vi "Process.vi"(8 "error in":errorcluster, 11 "EmbeddedMainUI":refnum<class "EmbeddedMainUI.lvclass">) -> (0 "error out":errorcluster, 3 "EmbeddedMainUI out":refnum<class "EmbeddedMainUI.lvclass">)   [LabVIEW 2016, in "EmbeddedMainUI.lvclass"]
doc: "---------------------------------------------------------------\nJKI State Machine Objects™\nhttp://jki.net/state-machine-objects/\nCopyright (C) 2005-2015, JKI <info@jki.net>\nALL RIGHTS RESERVEDJKI State Machine Objects (SMO) 1.0.0.5\nJKI - JKI\nCopyright (c) 2016, JKI"
uses:
  EmbeddedMainUI.lvclass
  C:/Program Files (x86)/National Instruments/LabVIEW 2016/vi.lib/JKI/JKI SMO/SMO/SMO.lvclass
  C:/Program Files (x86)/National Instruments/LabVIEW 2016/vi.lib/JKI/JKI SMO/SMO.UI/SMO.UI.lvclass
  <vilib>/JKI/JKI SMO/SMO/Typedefs/Parent Call--Enum.ctl
  <vilib>/Levylab/Embedded SMO UI/EmbeddedSMO.lvclass
  <vilib>/JKI/JKI SMO/SMO.UI/SMO.UI.lvclass
  <vilib>/JKI/JKI SMO/SMO/SMO.lvclass
panel:
  in  "Right Ring":u16(ring) items=["State One"]
  in  "Left Ring":u16(ring) items=["Mock1", "Mock2", "Mock3"]
  # "For instructions on how to use the JKI State Machine Objects, examples and video tutorials, visit:\nhttp://jki.net/state-machine-objects/\n\nJKI State Machine Objects™\nhttp://jki.net/state-machine-objects/\nCopyright (C) 2005-2015, JKI <info@jki.net>\nALL RIGHTS RESERVED"
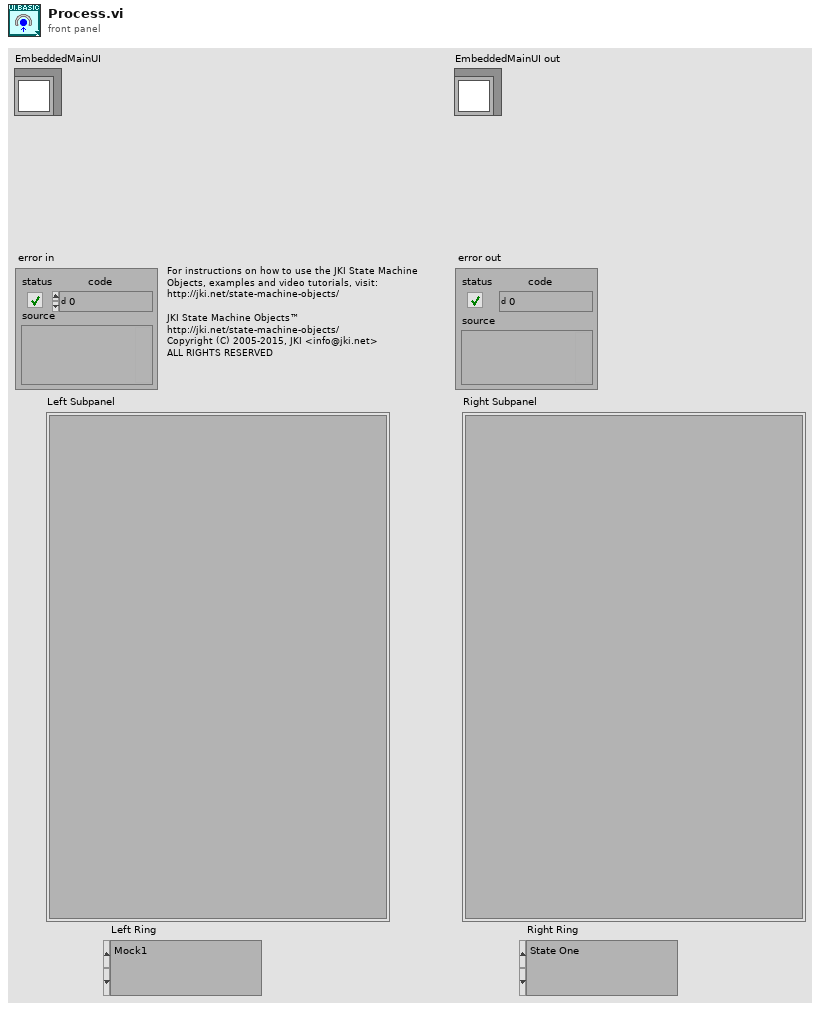
[diagram p1: front panel]
types:
  T1 = typedef "SMO.lvclass/Parent Call--Enum.ctl" = enum16{"Allows parent to run", "Does not request parent to run"}
  T2 = enum32{"invalid app kind", "Development System", "Run Time System", "Student Edition", "Embedded LabVIEW", "Evaluation", "Custom"}
  T3 = enum32{"Invalid", "Standard", "Closed", "Hidden", "Minimized", "Maximized"}
  T4 = cluster{"Core":cluster{"Current VI Reference":refnum<vi>, "Close Panel on Exit?":bool, "error":errorcluster}, "Self Reference":refnum<class "EmbeddedMainUI.lvclass">, "Right Subpanel":refnum<vi>, "Left Subpanel":refnum<vi>, "Left Ring":refnum<vi>, "Right Ring":refnum<vi>}
  T5 = cluster{"Current VI Reference":refnum<vi>, "Close Panel on Exit?":bool, "error":errorcluster}
  T6 = typedef "SMO.lvclass/Protected Events.ctl" = cluster{"StopProcesses":refnum<user-event>, "AbortProcesses":refnum<user-event>, "Config Changed":refnum<user-event>, "Dependency":refnum<user-event>}
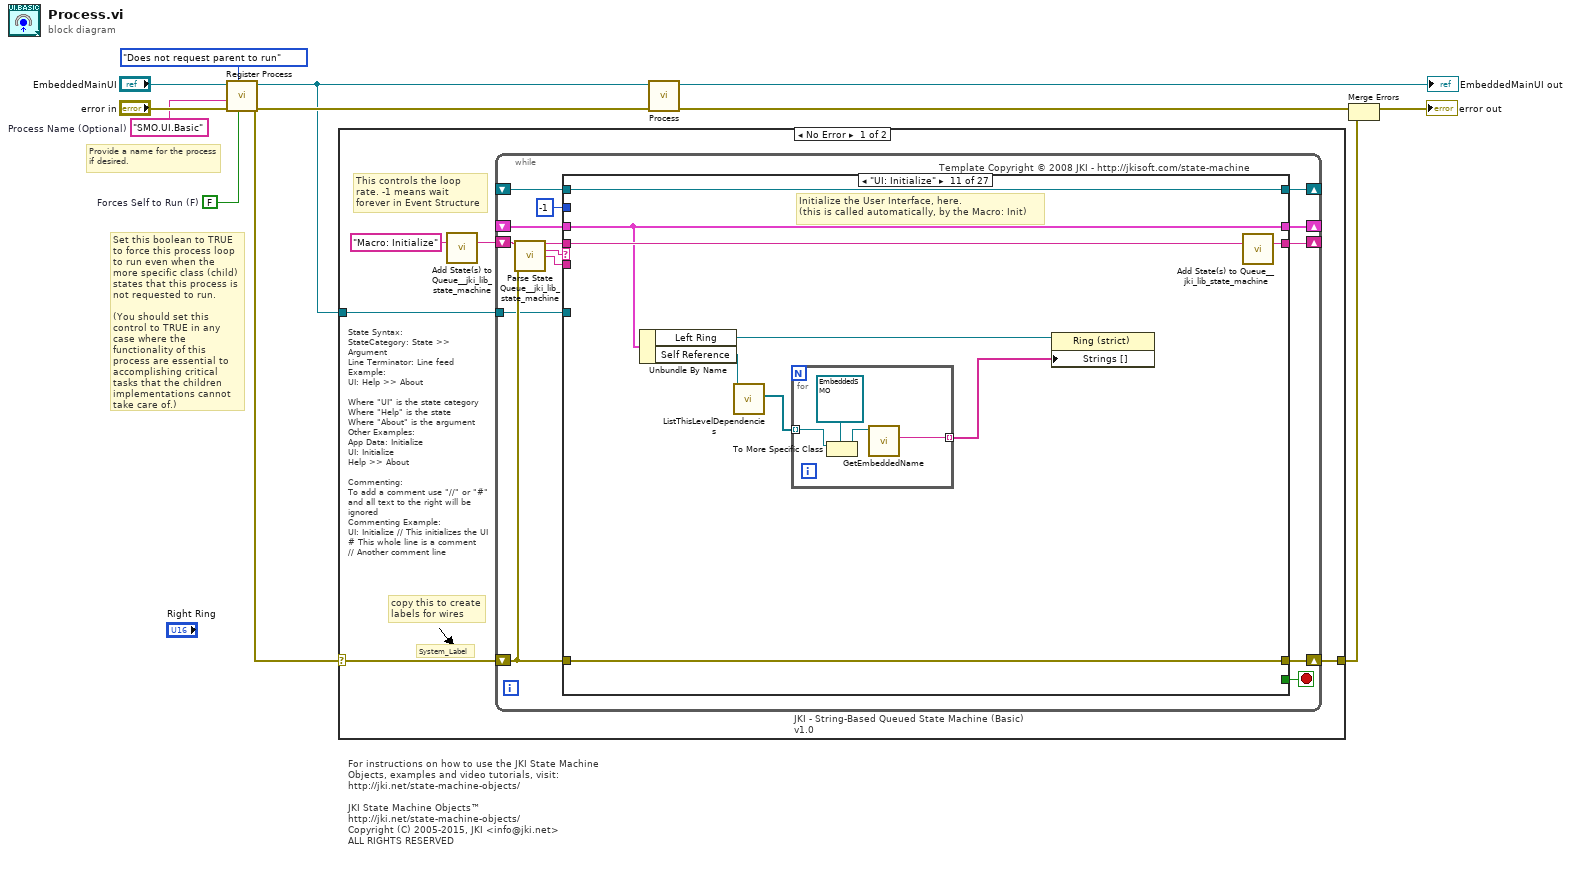
[diagram p0: block diagram]
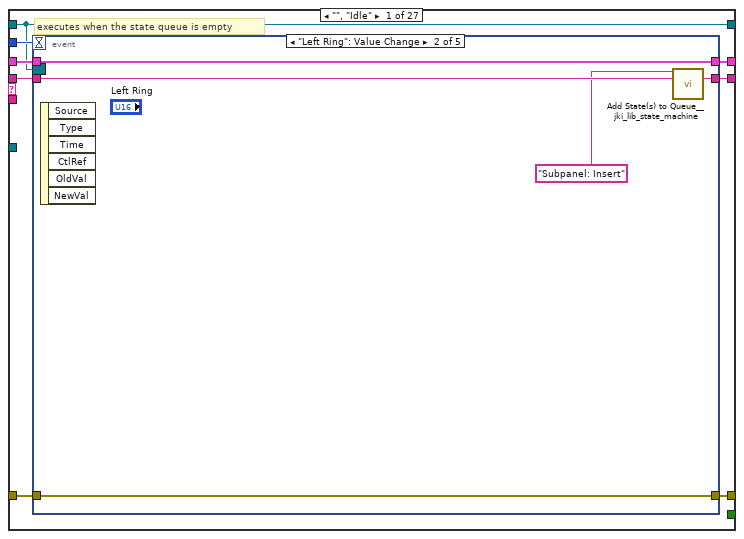
[diagram p2: hidden frame]
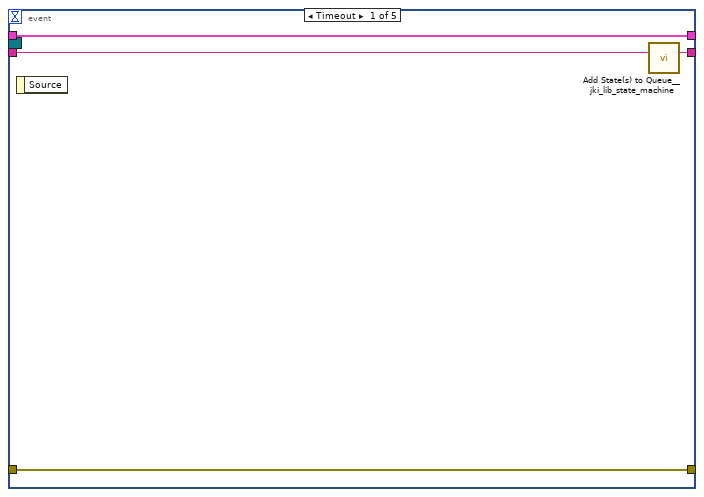
[diagram p3: hidden frame]
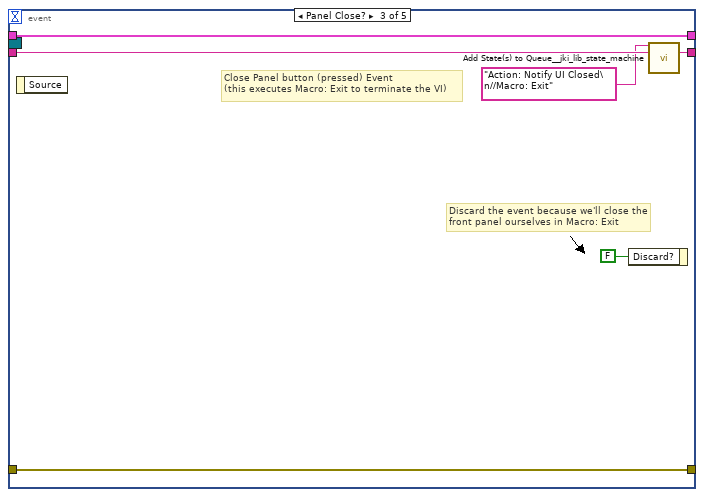
[diagram p4: hidden frame]
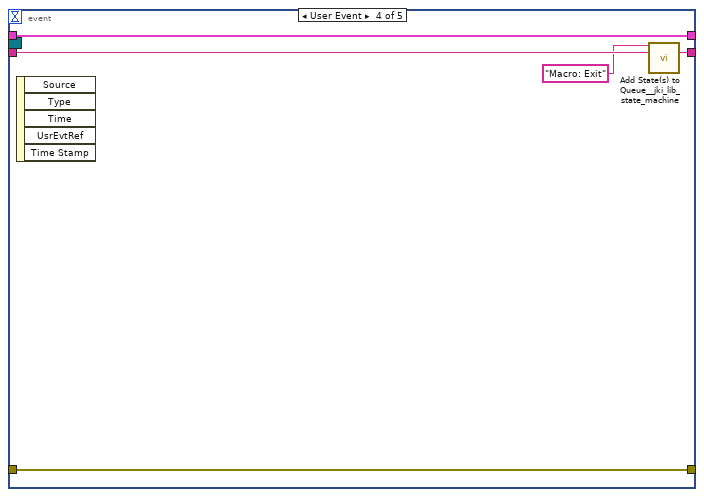
[diagram p5: hidden frame]
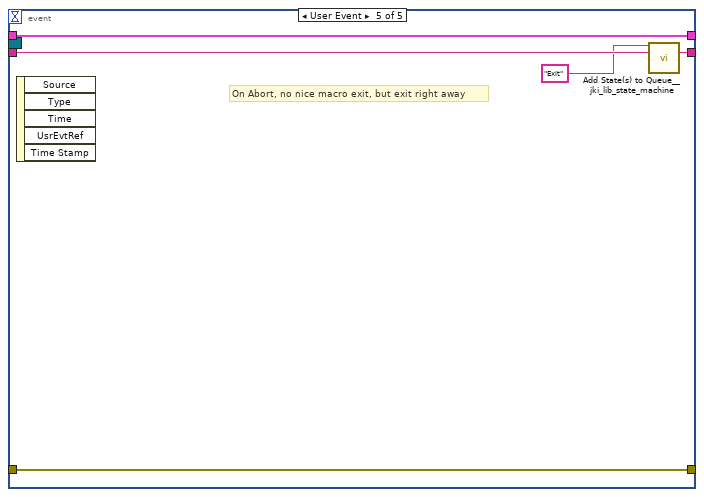
[diagram p6: hidden frame]
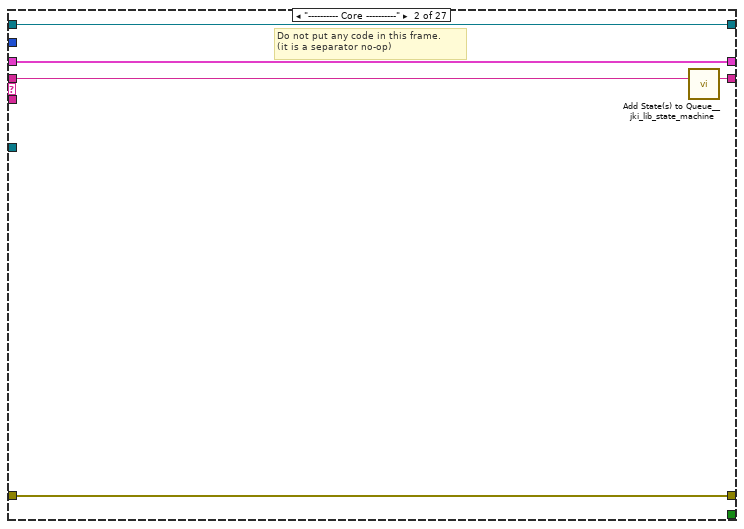
[diagram p7: hidden frame]
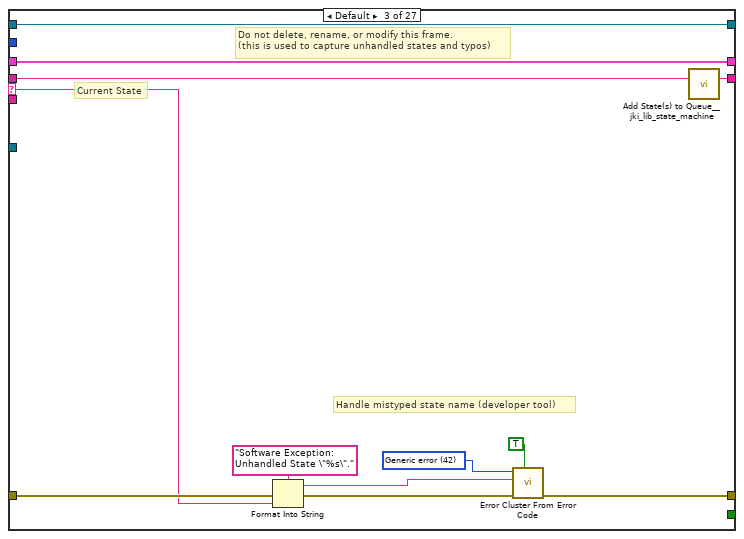
[diagram p8: hidden frame]
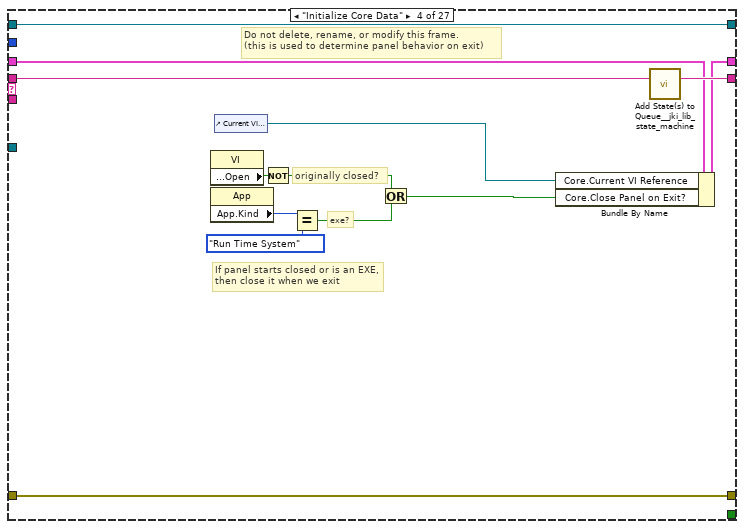
[diagram p9: hidden frame]
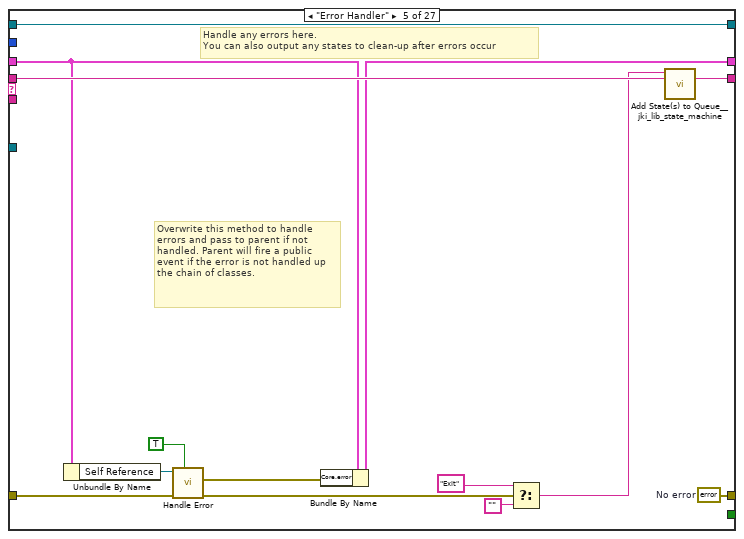
[diagram p10: hidden frame]
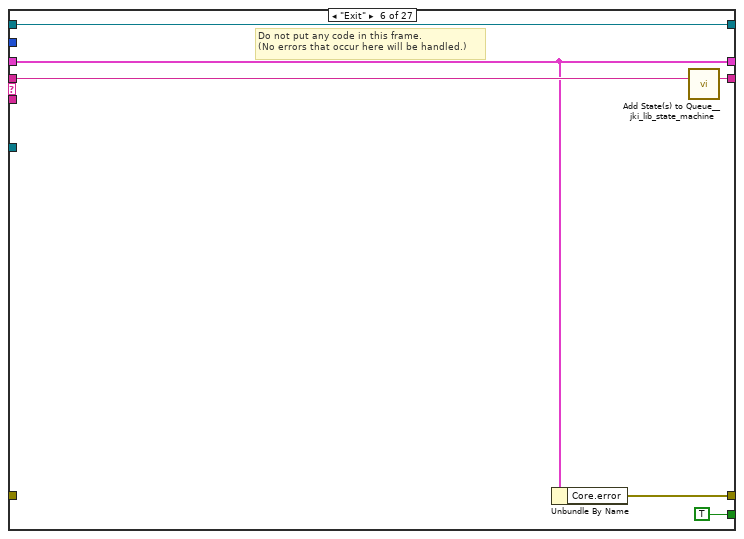
[diagram p11: hidden frame]
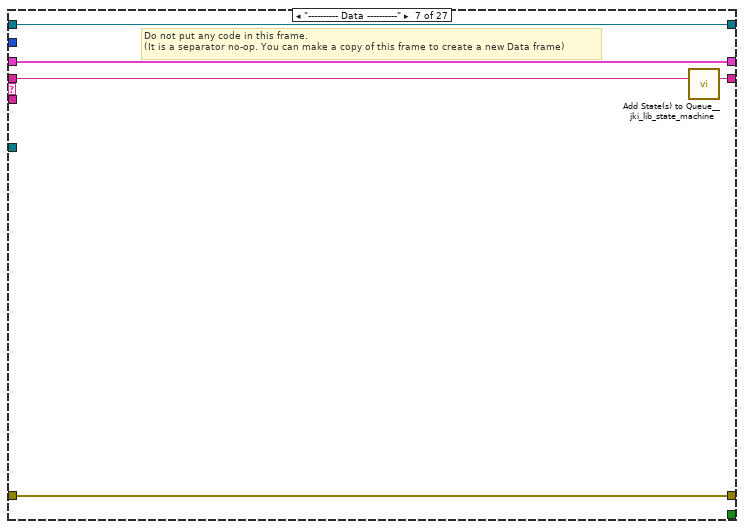
[diagram p12: hidden frame]
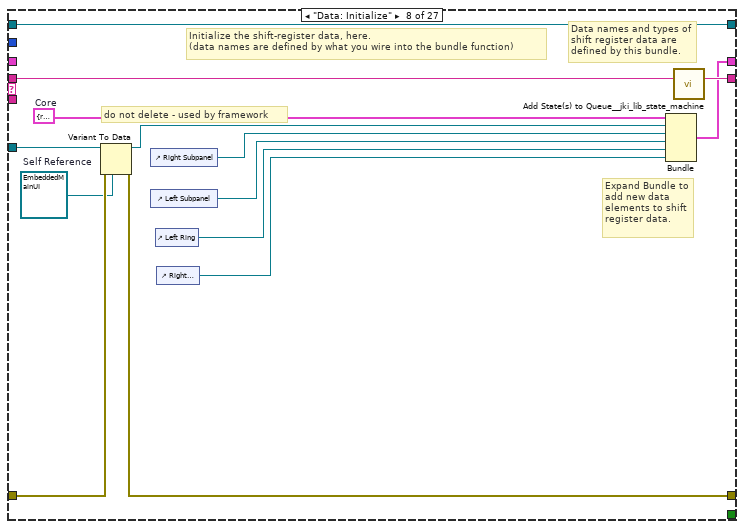
[diagram p13: hidden frame]
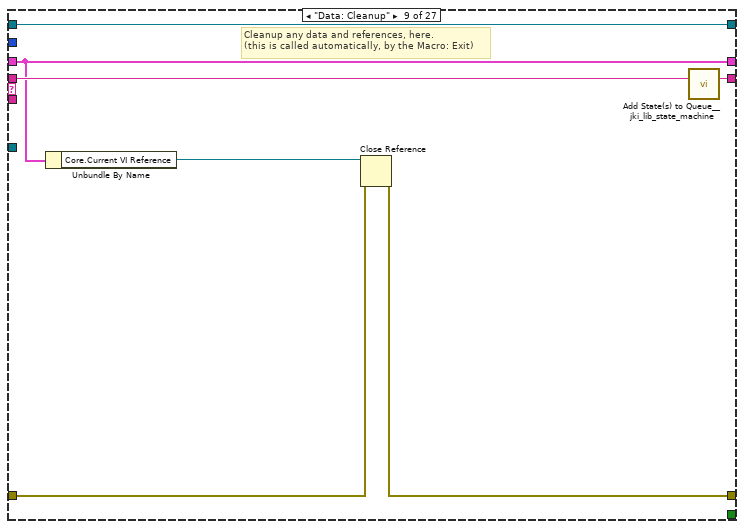
[diagram p14: hidden frame]
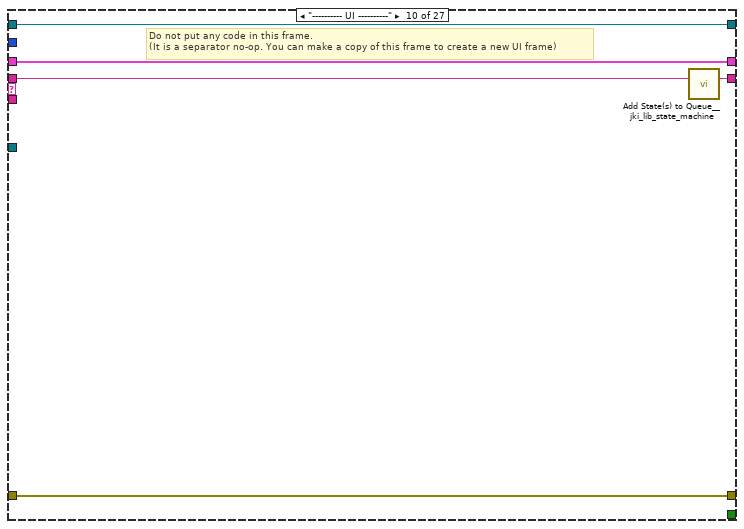
[diagram p15: hidden frame]
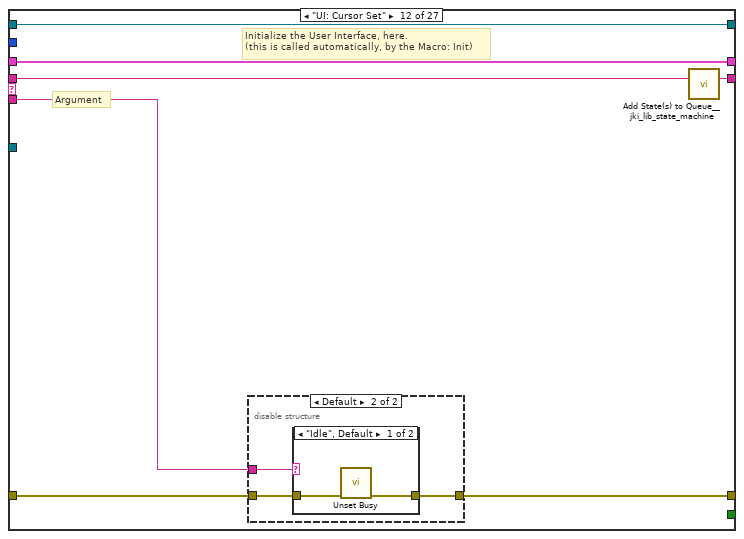
[diagram p16: hidden frame]
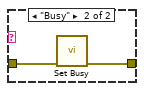
[diagram p18: hidden frame]
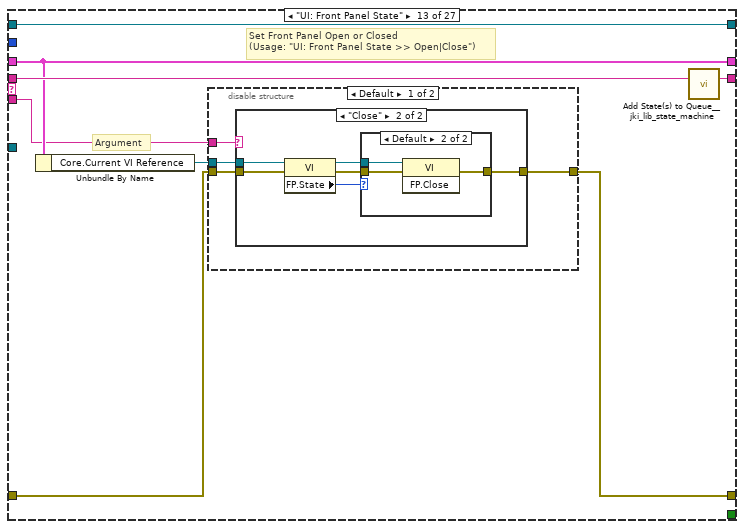
[diagram p19: hidden frame]
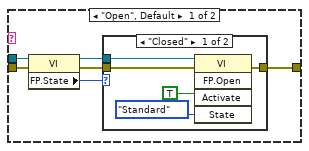
[diagram p20: hidden frame]
diagram:
  w2 = FALSE  # Forces Self to Run (F)
  w1 = "SMO.UI.Basic"  # Process Name (Optional)
  # "Provide a name for the process\nif desired."
  # "Set this boolean to TRUE to force this process loop to run even when the more specific class (child) states that this process is not requested to run.\n\n(You should set this control to TRUE in any case where the functionality of this process are essential to accomplishing critical tasks that the children implementations cannot take care of.)"
  # "For instructions on how to use the JKI State Machine Objects, examples and video tutorials, visit:\nhttp://jki.net/state-machine-objects/\n\nJKI State Machine Objects™\nhttp://jki.net/state-machine-objects/\nCopyright (C) 2005-2015, JKI <info@jki.net>\nALL RIGHTS RESERVED"
  n1 = call <vilib>:"Register Process.vi"("Forces Self to Run (F)"=w2, "Parent Call"=Parent_Call--Enum."Does not request parent to run", "error in (no error)"="error in", "Process Name (optional)"=w1, "SMO"="EmbeddedMainUI") -> ("error out"=w8:errorcluster, "SMO out"=w7:refnum<class "EmbeddedMainUI.lvclass">)  [unwired: 5 in]
  n2 = case shown="No Error" w8 {
    selector: w8 -> [w13 w320]
    tunnel: w7 -> [w14 _]
    tunnel: [w12 w320] -> w4
    frame No Error {
      # "State Syntax:\nStateCategory: State >> Argument\nLine Terminator: Line feed\nExample:\nUI: Help >> About\n\nWhere \"UI\" is the state category\nWhere \"Help\" is the state\nWhere \"About\" is the argument\nOther Examples:\nApp Data: Initialize\nUI: Initialize\nHelp >> About\n\nCommenting:\nTo add a comment use \"//\" or \"#\" and all text to the right will be ignored\nCommenting Example:\nUI: Initialize // This initializes the UI\n# This whole line is a comment\n// Another comment line"
      # "copy this to create labels for wires"
      # "This controls the loop rate. -1 means wait forever in Event Structure"
      # "System_Label"
      n3 = call <vilib>:"Add State(s) to Queue__jki_lib_state_machine.vi"("State(s) in (\"\")"="Macro: Initialize") -> ("States Out"=w16:string)  [unwired: 14 in]
      n4 = while "JKI - String-Based Queued State Machine (Basic) v1.0" {
        shift-right: [w23] -> _
        shift-left: _ -> [w22]
        shift-right: [w26] -> w12
        shift-left: w13 -> [w20]
        shift-right: [w25] -> _
        shift-left: w16 -> [w27]
        tunnel: w14 -> [w19]
        shift-right: [w18] -> _
        shift-left: _ -> [w17]
        stop <- w24 stop-if-true
        # "Template Copyright © 2008 JKI - http://jkisoft.com/state-machine"
        n5 = call <vilib>:"Parse State Queue__jki_lib_state_machine.vi"("State Queue"=w27, "Error In (no error)"=w20) -> ("Remaining States"=w29:string, "Current State"=w30:string, "Arguments"=w28:string)  [unwired: 11 in]
        n6 = case shown="\"UI: Initialize\"" w30 {
          selector: w30 -> [_ _ w70 _ _ _ _ _ _ _ _ _ _ _ _ _ _ _ _ _ _ _ _ _ _ _ _]
          tunnel: w29 -> [w38 w68 w74 w93 w107 w113 w118 w132 w139 w144 w153 w164 w180 w212 w221 w235 w240 w251 w256 w266 w272 w279 w286 w293 w298 w311 w319]
          tunnel: w28 -> [_ _ _ _ _ _ _ _ _ _ _ w158 w174 _ _ _ _ _ _ _ _ _ _ _ _ _ _]
          tunnel: w22 -> [w36 w65 w72 w84 w96 w109 w115 _ w134 w141 w149 w162 w176 w209 w217 w226 w237 w248 w253 w264 w270 w275 w282 w289 w295 w307 w316]
          tunnel: [w35 w66 w76 w90 w98 w108 w116 w128 w135 w142 w151 w159 w177 w210 w219 w233 w238 w242 w254 w258 w267 w276 w280 w290 w294 w308 w315] -> w26
          tunnel: w20 -> [w34 w66 w75 w90 w103 _ w116 w129 w136 w142 w151 w160 w178 w210 w219 w233 w238 w243 w254 w260 w268 w276 w281 w290 w294 w308 w315]
          tunnel: [w37 w67 w73 w92 w106 w112 w117 w131 w138 w143 w152 w163 w179 w211 w220 w234 w239 w250 w255 w265 w271 w278 w285 w292 w297 w310 w318] -> w25
          tunnel: [_ _ _ _ _ TRUE _ _ _ _ _ _ _ _ _ _ _ _ _ _ _ _ _ _ _ _ _] -> w24
          tunnel: [w33 w65 w72 w91 w95 w109 w115 w130 w134 w141 w149 w162 w176 w209 w217 w226 w237 w248 w253 w264 w270 w274 w282 w288 w295 w307 w316] -> w23
          tunnel: -1 ("Timeout") -> [w32 _ _ _ _ _ _ _ _ _ _ _ _ _ _ _ _ _ _ _ _ _ _ _ _ _ _]
          tunnel: w19 -> [_ _ _ _ _ _ _ w126 _ _ _ _ _ _ _ _ _ _ _ _ _ _ _ _ _ _ _]
          tunnel: [w31 w64 w69 w81 w105 w110 w114 w124 w133 w140 w150 w161 w173 w208 w218 w227 w236 w249 w252 w263 w269 w277 w284 w291 w296 w309 w317] -> w18
          tunnel: w17 -> [w31 w64 w69 w81 w105 w110 w114 w124 w133 w140 w150 w161 w173 w208 w218 w227 w236 w249 w252 _ w269 w277 w284 w291 w296 w309 w317]
          frame "", "Idle" {
            # "executes when the state queue is empty"
            n7 = event shown="[1] \"Left Ring\": Value Change" {
              selector: w31 -> [_ _ _ _ _]
              dyn-events: _ -> [_ _ _ _ _]
              timeout: w32 -> [_ _ _ _ _]
              tunnel: w38 -> [w42 w47 w53 w58 w63]
              tunnel: [w41 w46 w52 w57 w62] -> w37
              tunnel: w36 -> [w39 w44 w49 w55 w60]
              tunnel: [w40 w45 w48 w56 w61] -> w35
              tunnel: w34 -> [w40 w45 w48 w56 w61]
              tunnel: [w39 w44 w49 w55 w60] -> w33
              event Timeout {
                n8 = event-data() -> ()  [unwired: 1 in, 1 out]
                n9 = call <vilib>:"Add State(s) to Queue__jki_lib_state_machine.vi"("State(s) in (\"\")"=w42) -> ("States Out"=w41:string)  [unwired: 14 in]
              }
              event "Left Ring": Value Change {
                n10 = event-data() -> ()  [unwired: 1 in, 6 out]
                n11 = call <vilib>:"Add State(s) to Queue__jki_lib_state_machine.vi"("State(s) in Front (\"\")"="Subpanel: Insert", "State(s) in (\"\")"=w47) -> ("States Out"=w46:string)  [unwired: 13 in]
              }
              event Panel Close? {
                # "Discard the event because we'll close the front panel ourselves in Macro: Exit"
                # "Close Panel button (pressed) Event\n(this executes Macro: Exit to terminate the VI)"
                n12 = event-data() -> ()  [unwired: 1 in, 1 out]
                n13 = event-data("Discard?"=FALSE) -> ()  [unwired: 1 in, 1 out]
                n14 = call <vilib>:"Add State(s) to Queue__jki_lib_state_machine.vi"("State(s) in Front (\"\")"="Action: Notify UI Closed\n//Macro: Exit", "State(s) in (\"\")"=w53) -> ("States Out"=w52:string)  [unwired: 13 in]
              }
              event User Event {
                n15 = event-data() -> ()  [unwired: 1 in, 5 out]
                n16 = call <vilib>:"Add State(s) to Queue__jki_lib_state_machine.vi"("State(s) in Front (\"\")"="Macro: Exit", "State(s) in (\"\")"=w58) -> ("States Out"=w57:string)  [unwired: 13 in]
              }
              event User Event {
                # "On Abort, no nice macro exit, but exit right away"
                n17 = event-data() -> ()  [unwired: 1 in, 5 out]
                n18 = call <vilib>:"Add State(s) to Queue__jki_lib_state_machine.vi"("State(s) in Front (\"\")"="Exit", "State(s) in (\"\")"=w63) -> ("States Out"=w62:string)  [unwired: 13 in]
              }
            }
          }
          frame "---------- Core ----------" {
            # "Do not put any code in this frame.\n(it is a separator no-op)"
            n19 = call <vilib>:"Add State(s) to Queue__jki_lib_state_machine.vi"("State(s) in (\"\")"=w68) -> ("States Out"=w67:string)  [unwired: 14 in]
          }
          frame Default {
            w79 = 42 items=["No error", "Argument error", "Memory is full", "Out of zone", "End of file", "File already open", "Generic file I/O error", "File not found", "File permission error", "Disk is full", "Duplicate path", "Too many files open", "System feature not enabled", "Resource file not found", "Cannot add resource", "Resource not found", "Image not found", "Image memory error", "Pen does not exist", "Config type invalid", "Config token not found", "Config parse error", "Config memory error", "Bad external code format", "Bad external code offset", "External code not present", "Null window", "Destroy window error", "Null menu", "Print aborted", "Bad print record", "Print driver error", "Windows error during printing", "Memory error during printing", "Print dialog error", "Generic print error", "Invalid device refnum", "Device not found", "Device parameter error", "Device unit error", "Cannot open device", "Device call aborted", "Generic error", "Cancelled by user", "Object ID too low", "Object ID too high", "Object not in heap", "Unknown heap", "Unknown object (invalid DefProc)", "Unknown object (DefProc not in table)", "Message out of range", "Invalid (null) method", "Unknown message", "Manager call not supported", "Bad address", "Network operation in progress", "Network operation timed out", "Connection is busy", "Network attribute not supported", "Network error", "Address in use", "System out of memory", "Connection aborted", "Connection refused", "Not connected", "Already connected", "Connection closed", "Initialization error (interapplication manager)", "Bad occurrence", "Wait on unbound occurrence handler", "Occurrence queue overflow", "Datalog type conflict", "Unused", "Unrecognized type (interapplication manager)", "Memory corrupt", "Failed to make temporary DLL", "Old CIN version", "Drag socket not found", "Failed to load drop-object", "Failed to register OLE object", "Failed to release OLE object", "Format specifier type mismatch", "Unknown format specifier", "Too few format specifiers", "Too many format specifiers", "Scan failed", "Newer CIN version", "Error converting to variant", "Runtime menu error", "Password tampered", "Variant attribute not found", "Incompatible variant data type", "Event data is not available", "Event Store is not present", "Occurrence is not found", "Event Queue is not created", "Event info is not available", "Refnum passed is NULL", "Error retrieving Class GUID", "Error retrieving CoClass GUID", "Error retrieving TypeLib GUID.", "Bad built application magic bytes.", "Specific driver is different from the specific driver associated with the Logical Name.", "There is no session opened to the class driver.", "Max Error", "MAX - Error with config objects", "MAX - Error loading configuration", "MAX - Group not supported"]
            # "Current State"
            # "Do not delete, rename, or modify this frame.\n(this is used to capture unhandled states and typos)"
            # "Handle mistyped state name (developer tool)"
            n20 = Format Into String(format string="Software Exception: Unhandled State \"%s\"." ("message"), error in=w75, w70) -> (resulting string=w78:string, error out=w77:errorcluster)  [unwired: 1 in]
            n21 = call <vilib>:"Error Cluster From Error Code.vi"("show call chain? (False)"=TRUE, "error in (no error)"=w77, "error message (\"\")"=w78, "error code (0)"=w79) -> ("error out"=w76:errorcluster)  [unwired: 5 in]
            n22 = call <vilib>:"Add State(s) to Queue__jki_lib_state_machine.vi"("State(s) in (\"\")"=w74) -> ("States Out"=w73:string)  [unwired: 14 in]
          }
          frame "Initialize Core Data" {
            # "Do not delete, rename, or modify this frame.\n(this is used to determine panel behavior on exit)"
            # "originally closed?"
            # "exe?"
            # "If panel starts closed or is an EXE, then close it when we exit"
            n23 = property class="VI"() -> ("Front Panel.Open"=w89:bool)  [unwired: 2 in, 2 out]
            n24 = property class="App"() -> ("App.Kind"=w88:T2)  [unwired: 2 in, 2 out]
            n25 = control-ref of="Current VI Reference"() -> (w82:refnum<vi>)
            n26 = Not(x=w89) -> (.not. x?=w86:bool)
            n27 = Equal?(x=w88, y=T2."Run Time System" ("Application:Kind")) -> (x = y?=w85:bool)
            n28 = Or(x=w86, y=w85) -> (x .or. y?=w83:bool)
            n29 = Bundle By Name(cluster=w84, "Core.Current VI Reference"=w82, "Core.Close Panel on Exit?"=w83) -> (w91:T4)
            n30 = call <vilib>:"Add State(s) to Queue__jki_lib_state_machine.vi"("State(s) in (\"\")"=w93) -> ("States Out"=w92:string)  [unwired: 14 in]
          }
          frame "Error Handler" {
            w98 = errorcluster {"status"=FALSE, "code"=0, "source"=""}  # No error
            # "Overwrite this method to handle errors and pass to parent if not handled. Parent will fire a public event if the error is not handled up the chain of classes."
            # "Handle any errors here.\nYou can also output any states to clean-up after errors occur"
            n31 = Unbundle By Name(w96) -> ("Self Reference"=w104:refnum<class "EmbeddedMainUI.lvclass">)
            n32 = call-dynamic "Handle Error.vi"("Stop on Unhandled Error (T)"=TRUE, "error in"=w103, "SMO"=w104) -> ("handling error"=w99:errorcluster, "Unhandled error"=w97:errorcluster)  [unwired: 6 in, 1 out]
            n33 = Bundle By Name(cluster=w96, "Core.error"=w97) -> (w95:T4)
            n34 = Select(t="Exit", s=w99, f="") -> (s? t:f=w100:string)
            n35 = call <vilib>:"Add State(s) to Queue__jki_lib_state_machine.vi"("State(s) in Front (\"\")"=w100, "State(s) in (\"\")"=w107) -> ("States Out"=w106:string)  [unwired: 13 in]
          }
          frame "Exit" {
            # "Do not put any code in this frame.\n(No errors that occur here will be handled.)"
            n36 = Unbundle By Name(w109) -> ("Core.error"=w108:errorcluster)
            n37 = call <vilib>:"Add State(s) to Queue__jki_lib_state_machine.vi"("State(s) in (\"\")"=w113) -> ("States Out"=w112:string)  [unwired: 14 in]
          }
          frame "---------- Data ----------" {
            # "Do not put any code in this frame.\n(It is a separator no-op. You can make a copy of this frame to create a new Data frame)"
            n38 = call <vilib>:"Add State(s) to Queue__jki_lib_state_machine.vi"("State(s) in (\"\")"=w118) -> ("States Out"=w117:string)  [unwired: 14 in]
          }
          frame "Data: Initialize" {
            w123 = T5 {"Current VI Reference"=refnum, "Close Panel on Exit?"=FALSE, "error"={"status"=FALSE, "code"=0, "source"=""}}  # Core
            w127 = refnum<class "EmbeddedMainUI.lvclass"> refnum  # Self Reference
            # "do not delete - used by framework"
            # "Expand Bundle to add new data elements to shift register data."
            # "Data names and types of shift register data are defined by this bundle."
            # "Initialize the shift-register data, here.\n(data names are defined by what you wire into the bundle function)"
            n39 = Variant To Data(error in=w129, type=w127, Variant=w126) -> (data=w125:refnum<class "EmbeddedMainUI.lvclass">, error out=w128:errorcluster)
            n40 = control-ref of="Right Subpanel"() -> (w122:refnum<vi>)
            n41 = control-ref of="Left Subpanel"() -> (w121:refnum<vi>)
            n42 = control-ref of="Left Ring"() -> (w120:refnum<vi>)
            n43 = control-ref of="Right Ring"() -> (w119:refnum<vi>)
            n44 = Bundle("Core"=w123, "Self Reference"=w125, "Right Subpanel"=w122, "Left Subpanel"=w121, "Left Ring"=w120, "Right Ring"=w119) -> (w130:T4)  [unwired: 1 in]
            n45 = call <vilib>:"Add State(s) to Queue__jki_lib_state_machine.vi"("State(s) in (\"\")"=w132) -> ("States Out"=w131:string)  [unwired: 14 in]
          }
          frame "Data: Cleanup" {
            # "Cleanup any data and references, here.\n(this is called automatically, by the Macro: Exit)"
            n46 = Unbundle By Name(w134) -> ("Core.Current VI Reference"=w137:refnum<vi>)
            n47 = Close Reference(reference=w137, error in (no error)=w136) -> (error out=w135:errorcluster)
            n48 = call <vilib>:"Add State(s) to Queue__jki_lib_state_machine.vi"("State(s) in (\"\")"=w139) -> ("States Out"=w138:string)  [unwired: 14 in]
          }
          frame "---------- UI ----------" {
            # "Do not put any code in this frame.\n(It is a separator no-op. You can make a copy of this frame to create a new UI frame)"
            n49 = call <vilib>:"Add State(s) to Queue__jki_lib_state_machine.vi"("State(s) in (\"\")"=w144) -> ("States Out"=w143:string)  [unwired: 14 in]
          }
          frame "UI: Initialize" {
            # "Initialize the User Interface, here.\n(this is called automatically, by the Macro: Init)"
            n50 = Unbundle By Name(w149) -> ("Left Ring"=w148:refnum<vi>, "Self Reference"=w147:refnum<class "EmbeddedMainUI.lvclass">)
            n51 = call <vilib>:"ListThisLevelDependencies.vi"("SMO in"=w147) -> ("[My Dependencies]"=w146:refnum<class "SMO.lvclass">[])  [unwired: 8 in, 2 out]
            n52 = for {
              tunnel: w146 -> [w156] mode=indexing
              tunnel: [w154] -> w145 mode=indexing
              n53 = To More Specific Class(target class=refnum<class "EmbeddedSMO.lvclass"> refnum ("EmbeddedSMO out"), reference=w156) -> (specific class reference=w155:refnum<class "EmbeddedSMO.lvclass">)  [unwired: 1 in, 1 out]
              n54 = call <vilib>:"GetEmbeddedName.vi"("EmbeddedSMO in"=w155) -> ("Name"=w154:string)  [unwired: 8 in, 2 out]
            }
            n55 = property class="Ring (strict)"(reference=w148, "Strings []"=w145) -> ()  [unwired: 1 in, 2 out]
            n56 = call <vilib>:"Add State(s) to Queue__jki_lib_state_machine.vi"("State(s) in (\"\")"=w153) -> ("States Out"=w152:string)  [unwired: 14 in]
          }
          frame "UI: Cursor Set" {
            # "Argument"
            # "Initialize the User Interface, here.\n(this is called automatically, by the Macro: Init)"
            n57 = disable-structure shown="Default" {
              disable-tunnel: w160 -> [w165 w168]
              disable-tunnel: [w165 w167] -> w159
              disable-tunnel: w158 -> [_ w166]
              frame condition #0 {
              }
              frame condition #1 (active) {
                n58 = case shown="\"Idle\", Default" w166 {
                  tunnel: w168 -> [w170 w172]
                  tunnel: [w169 w171] -> w167
                  frame "Idle", Default {
                    n59 = call <vilib>:"Unset Busy.vi"("error in (no error)"=w170) -> ("error out"=w169:errorcluster)  [unwired: 10 in]
                  }
                  frame "Busy" {
                    n60 = call <vilib>:"Set Busy.vi"("error in (no error)"=w172) -> ("error out"=w171:errorcluster)  [unwired: 9 in, 1 out]
                  }
                }
              }
            }
            n61 = call <vilib>:"Add State(s) to Queue__jki_lib_state_machine.vi"("State(s) in (\"\")"=w164) -> ("States Out"=w163:string)  [unwired: 14 in]
          }
          frame "UI: Front Panel State" {
            # "Argument"
            # "Set Front Panel Open or Closed\n(Usage: \"UI: Front Panel State >> Open|Close\")"
            n62 = Unbundle By Name(w176) -> ("Core.Current VI Reference"=w175:refnum<vi>)
            n63 = disable-structure shown="Default" {
              disable-tunnel: w178 -> [w184 w207]
              disable-tunnel: [w183 w207] -> w177
              disable-tunnel: w175 -> [w182 _]
              disable-tunnel: w174 -> [w181 _]
              frame condition #0 (active) {
                n64 = case shown="\"Close\"" w181 {
                  tunnel: w184 -> [w188 w201]
                  tunnel: [w190 w202] -> w183
                  tunnel: w182 -> [w189 w199]
                  frame "Open", Default {
                    n65 = property class="VI"(reference=w189, error in=w188) -> (reference out=w186:refnum<vi>, error out=w187:errorcluster, "FP.State"=w185:T3)
                    n66 = case shown="\"Closed\"" w185 {
                      tunnel: [w193 w196] -> w190
                      tunnel: w187 -> [w192 w196]
                      tunnel: w186 -> [w191 _]
                      frame "Closed" {
                        n67 = invoke class="VI" method="FP.Open"(reference=w191, error in=w192, "Activate"=TRUE, "State"=T3."Standard") -> (error out=w193:errorcluster)  [unwired: 1 in, 4 out]
                      }
                      frame Default {
                      }
                    }
                  }
                  frame "Close" {
                    n68 = property class="VI"(reference=w199, error in=w201) -> (reference out=w198:refnum<vi>, error out=w200:errorcluster, "FP.State"=w197:T3)
                    n69 = case shown="Default" w197 {
                      tunnel: [w203 w206] -> w202
                      tunnel: w200 -> [w203 w205]
                      tunnel: w198 -> [_ w204]
                      frame "Invalid", "Closed" {
                      }
                      frame Default {
                        n70 = invoke class="VI" method="FP.Close"(reference=w204, error in=w205) -> (error out=w206:errorcluster)  [unwired: 1 in, 2 out]
                      }
                    }
                  }
                }
              }
              frame condition #1 {
              }
            }
            n71 = call <vilib>:"Add State(s) to Queue__jki_lib_state_machine.vi"("State(s) in (\"\")"=w180) -> ("States Out"=w179:string)  [unwired: 14 in]
          }
          frame "---------- Macro ----------" {
            # "Do not put any code in this frame.\n(It is a separator no-op. You can make a copy of this frame to create a new Macro frame)"
            n72 = call <vilib>:"Add State(s) to Queue__jki_lib_state_machine.vi"("State(s) in (\"\")"=w212) -> ("States Out"=w211:string)  [unwired: 14 in]
          }
          frame "Macro: Initialize" {
            w215 = "UI: Initialize\n//UI: Front Panel State >> Open\nSubpanel: Start\nSubpanel: Insert"  # UI: Initialize //UI: Front Panel State >> Open Subpanel: Start Subpanel: Insert
            # "Initialization Macro\n(This is called once, when the VI starts)"
            n73 = call <vilib>:"Add State(s) to Queue__jki_lib_state_machine.vi"("State(s) in Front (\"\")"="Data: Initialize\nInitialize Core Data\nEvents: Register", "State(s) in (\"\")"="Process: Sync", "State(s) at Back (\"\")"=w215) -> ("States Out"=w214:string)  [unwired: 12 in]
            n74 = call <vilib>:"Add State(s) to Queue__jki_lib_state_machine.vi"("State(s) in Front (\"\")"=w214, "State(s) in (\"\")"=w221) -> ("States Out"=w220:string)  [unwired: 13 in]
          }
          frame "Macro: Exit" {
            # "Exit Macro\n(This is called once, when the VI exits)"
            n75 = Unbundle By Name(w226) -> ("Core.Close Panel on Exit?"=w232:bool)
            n76 = Select(t="//UI: Front Panel State >> Close", s=w232, f="") -> (s? t:f=w229:string)
            n77 = call <vilib>:"Add State(s) to Queue__jki_lib_state_machine.vi"("State(s) in Front (\"\")"="Subpanel: Stop\nData: Cleanup\nEvents: Unregister", "State(s) in (\"\")"="Process: Sync", "State(s) at Back (\"\")"="Exit") -> ("States Out"=w223:string)  [unwired: 12 in]
            n78 = call <vilib>:"Add State(s) to Queue__jki_lib_state_machine.vi"("State(s) in (\"\")"=w229, "State(s) at Back (\"\")"=w223) -> ("States Out"=w228:string)  [unwired: 13 in]
            n79 = call <vilib>:"Add State(s) to Queue__jki_lib_state_machine.vi"("State(s) in Front (\"\")"=w228, "State(s) in (\"\")"=w235) -> ("States Out"=w234:string)  [unwired: 13 in]
          }
          frame "---------- Process ----------" {
            # "Template Separator\n(You can make a copy of, or modify, this frame)"
            n80 = call <vilib>:"Add State(s) to Queue__jki_lib_state_machine.vi"("State(s) in (\"\")"=w240) -> ("States Out"=w239:string)  [unwired: 14 in]
          }
          frame "Process: Sync" {
            n81 = Unbundle By Name(w248) -> ("Self Reference"=w244:refnum<class "EmbeddedMainUI.lvclass">)
            n82 = call <vilib>:"WaitOnProcessSync.vi"("error in (no error)"=w243, "SMO"=w244) -> ("error out"=w242:errorcluster, "Don't run?"=w247:bool)  [unwired: 7 in, 1 out]
            n83 = Select(t="Data: Cleanup\nEvents: Unregister\nExit", s=w247, f="") -> (s? t:f=w241:string)
            n84 = call <vilib>:"Add State(s) to Queue__jki_lib_state_machine.vi"("State(s) in Front (\"\")"=w241, "State(s) in (\"\")"=w251) -> ("States Out"=w250:string)  [unwired: 13 in]
          }
          frame "---------- Events ----------" {
            # "Template Separator\n(You can make a copy of, or modify, this frame)"
            n85 = call <vilib>:"Add State(s) to Queue__jki_lib_state_machine.vi"("State(s) in (\"\")"=w256) -> ("States Out"=w255:string)  [unwired: 14 in]
          }
          frame "Events: Register" {
            # "Expand to add\nmore events"
            # "Base Class Protected Events"
            n86 = Unbundle By Name(w264) -> ("Self Reference"=w261:refnum<class "EmbeddedMainUI.lvclass">)
            n87 = call <vilib>:"GetProtectedEvents.vi"("SMO"=w261) -> ("error out"=w257:errorcluster, "SMO Protected Events"=w262:T6)  [unwired: 8 in, 1 out]
            n88 = register-events(w262) -> (reference out=w263:refnum<event-registration>, error out=w259:errorcluster)  [unwired: 2 in]
            n89 = Merge Errors(w260, w259, w257) -> (w258:errorcluster)
            n90 = call <vilib>:"Add State(s) to Queue__jki_lib_state_machine.vi"("State(s) in (\"\")"=w266) -> ("States Out"=w265:string)  [unwired: 14 in]
          }
          frame "Events: Unregister" {
            n91 = Unregister For Events(event registration refnum=w269, error in=w268) -> (error out=w267:errorcluster)
            n92 = call <vilib>:"Add State(s) to Queue__jki_lib_state_machine.vi"("State(s) in (\"\")"=w272) -> ("States Out"=w271:string)  [unwired: 14 in]
          }
          frame "---------- Action ----------" {
            n93 = Unbundle By Name(w275) -> ("Self Reference"=w273:refnum<class "EmbeddedMainUI.lvclass">)
            n94 = Bundle By Name(cluster=w275, "Self Reference"=w273) -> (w274:T4)
            n95 = call <vilib>:"Add State(s) to Queue__jki_lib_state_machine.vi"("State(s) in (\"\")"=w279) -> ("States Out"=w278:string)  [unwired: 14 in]
          }
          frame "Action: Notify UI Closed" {
            # "Notify that the UI has been closed"
            n96 = Unbundle By Name(w282) -> ("Self Reference"=w283:refnum<class "EmbeddedMainUI.lvclass">)
            n97 = call <vilib>:"Hide.vi"("error in (no error)"=w281, "SMO.UI"=w283) -> ("error out"=w280:errorcluster)  [unwired: 8 in, 1 out]
            n98 = call <vilib>:"Add State(s) to Queue__jki_lib_state_machine.vi"("State(s) in (\"\")"=w286) -> ("States Out"=w285:string)  [unwired: 14 in]
          }
          frame "---------- Subpanel ----------" {
            n99 = Unbundle By Name(w289) -> ("Self Reference"=w287:refnum<class "EmbeddedMainUI.lvclass">)
            n100 = Bundle By Name(cluster=w289, "Self Reference"=w287) -> (w288:T4)
            n101 = call <vilib>:"Add State(s) to Queue__jki_lib_state_machine.vi"("State(s) in (\"\")"=w293) -> ("States Out"=w292:string)  [unwired: 14 in]
          }
          frame "Subpanel: Start" {
            n102 = call <vilib>:"Add State(s) to Queue__jki_lib_state_machine.vi"("State(s) in (\"\")"=w298) -> ("States Out"=w297:string)  [unwired: 14 in]
          }
          frame "Subpanel: Insert" {
            n103 = Unbundle By Name(w307) -> ("Left Subpanel"=w299:refnum<vi>, "Self Reference"=w306:refnum<class "EmbeddedMainUI.lvclass">, "Left Ring"=w303:refnum<vi>)
            n104 = property class="Ring (strict)"(reference=w303) -> ("Value"=w301:u16)  [unwired: 1 in, 2 out]
            n105 = call <vilib>:"ListThisLevelDependencies.vi"("SMO in"=w306) -> ("[My Dependencies]"=w304:refnum<class "SMO.lvclass">[])  [unwired: 8 in, 2 out]
            n106 = for {
              tunnel: refnum<class "EmbeddedSMO.lvclass"> refnum ("EmbeddedSMO") -> [w314]
              tunnel: w304 -> [w313] mode=indexing
              tunnel: [w312] -> w302 mode=indexing
              n107 = To More Specific Class(target class=w314, reference=w313) -> (specific class reference=w312:refnum<class "EmbeddedSMO.lvclass">)  [unwired: 1 in, 1 out]
            }
            n108 = Index Array(array=w302, index=w301) -> (element=w300:refnum<class "EmbeddedSMO.lvclass">)
            n109 = call <vilib>:"Embed_Show.vi"("Sub Panel"=w299, "EmbeddedSMO in"=w300) -> ()  [unwired: 8 in, 2 out]
            n110 = call <vilib>:"Add State(s) to Queue__jki_lib_state_machine.vi"("State(s) in (\"\")"=w311) -> ("States Out"=w310:string)  [unwired: 14 in]
          }
          frame "Subpanel: Stop" {
            n111 = call <vilib>:"Add State(s) to Queue__jki_lib_state_machine.vi"("State(s) in (\"\")"=w319) -> ("States Out"=w318:string)  [unwired: 14 in]
          }
        }
      }
    }
    frame Error {
    }
  }
  n112 = call-parent "Process.vi"("error in (no error)"=w8, "SMO.UI"=w7) -> ("error out"=w5:errorcluster, "SMO.UI out"=→"EmbeddedMainUI out":refnum<class "EmbeddedMainUI.lvclass">)  [unwired: 8 in]
  n113 = Merge Errors(w5, w4) -> (→"error out":errorcluster)
